vi "Write TEC SP.vi"(8 "error in (no error)":errorcluster, 10 "TEC SP":sgl[](array[numeric]), 11 "Set TEC SP MSG in":refnum<class "Set TEC SP MSG.lvclass">) -> (0 "error out":errorcluster, 3 "Set TEC SP MSG out":refnum<class "Set TEC SP MSG.lvclass">)   [LabVIEW 2014, in "Set TEC SP MSG.lvclass"]
uses:
  Set TEC SP MSG.lvclass
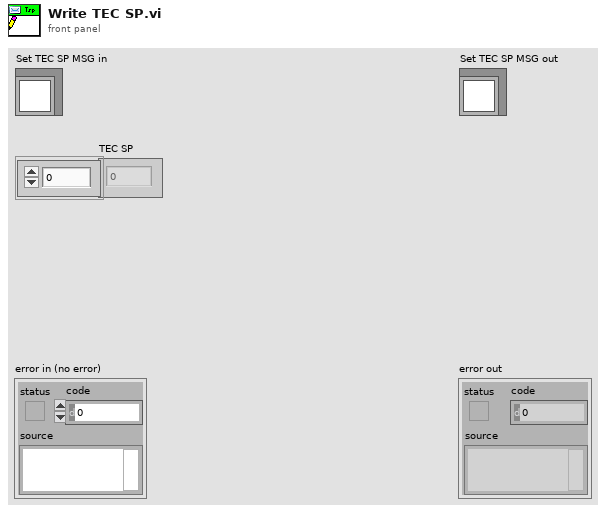
[diagram p1: front panel]
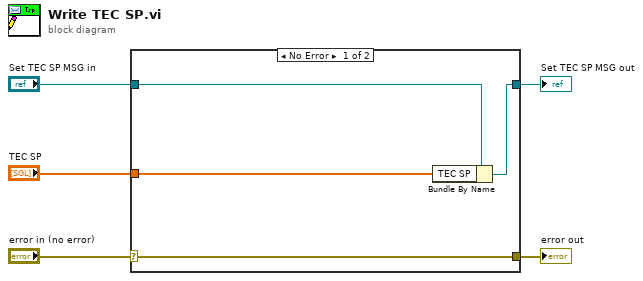
[diagram p0: block diagram]
diagram:
  n1 = case shown="No Error" "error in (no error)" {
    selector: "error in (no error)" -> [w9 w10]
    tunnel: [w9 w10] -> w4
    tunnel: [w7 w11] -> w2
    tunnel: "Set TEC SP MSG in" -> [w8 w11]
    tunnel: "TEC SP" -> [w6 _]
    frame No Error {
      n2 = Bundle By Name(cluster=w8, "TEC SP"=w6) -> (w7:refnum<class "Set TEC SP MSG.lvclass">)
    }
    frame Error {
    }
  }
  "error out" <- w4
  "Set TEC SP MSG out" <- w2
